vi "通信原理实验任务 1_3何德轩.vi"() -> ()   [LabVIEW 2018]
uses:
  <vilib>/measure/NI_MABase.lvlib
panel:
  out "波形图 2":waveform(dbl)(graph)
  out "波形图":waveform(dbl)[](graph)
  in  "噪声":cluster{"An":dbl}={"An"=2.0}
  in  "信号":cluster{"Fc":dbl, "Ac":dbl}={"Fc"=1.0, "Ac"=10.0}
  in  "采样参数":cluster{"Fs":dbl, "采样数":dbl}={"Fs"=6.0, "采样数"=18.0}
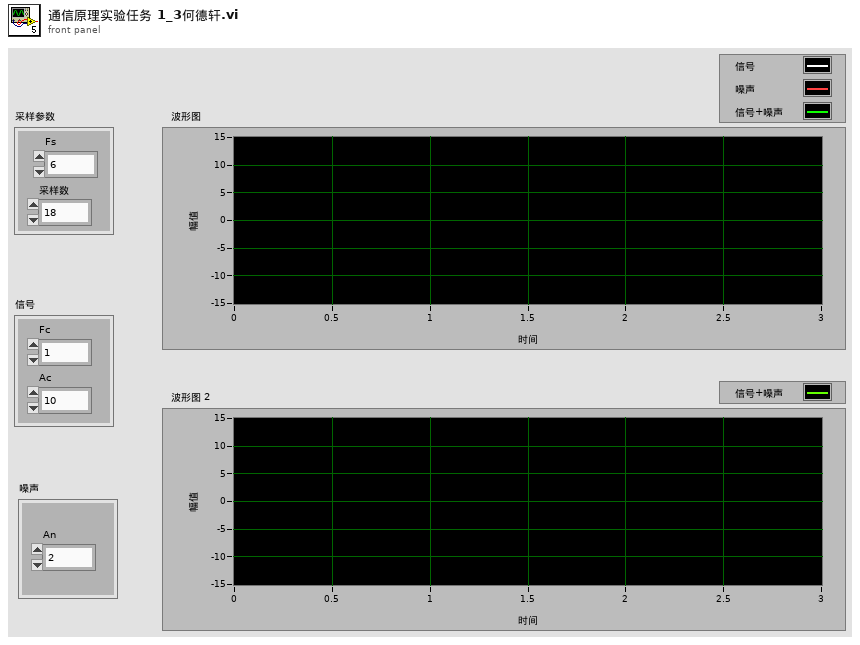
[diagram p1: front panel]
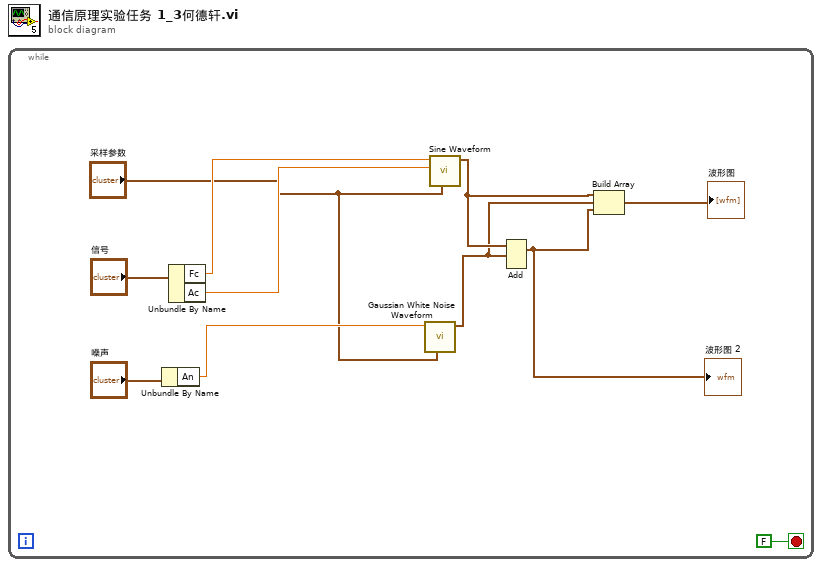
[diagram p0: block diagram]
diagram:
  n1 = while {
    stop <- FALSE stop-if-true
    n2 = Unbundle By Name("噪声") -> ("An"=w7:dbl)
    n3 = Unbundle By Name("信号") -> ("Fc"=w6:dbl, "Ac"=w5:dbl)
    n4 = call <vilib>:"Gaussian White Noise Waveform.vi"("sampling info"="采样参数", "standard deviation"=w7) -> ("signal out"=w2:waveform(dbl))  [unwired: 8 in, 1 out]
    n5 = call <vilib>:"Sine Waveform.vi"("sampling info"="采样参数", "amplitude"=w5, "frequency"=w6) -> ("signal out"=w3:waveform(dbl))  [unwired: 7 in, 1 out]
    n6 = Add(1:w2, 2:w3) -> (0:w10:waveform(dbl))  [unwired: 1 in, 1 out]
    "波形图 2" <- w10
    n7 = Build Array(w3, w2, w10) -> (→"波形图":waveform(dbl)[])
  }
